vi "Vision Processing.vi"(4 "error in (no error)":errorcluster, 7 "Image Size":T1=enum."320x240") -> ()   [LabVIEW 2016]
doc: "This VI runs in parallel to other tasks. It gets images from the camera, processes them for color or shape and use that information to affect robot behavior."
uses:
  <vilib>/Rock Robotics/WPI/Camera/WPI_CameraImageSize.ctl
  <vilib>/Rock Robotics/WPI/Camera/WPI_CameraWhite Balance Values.ctl
  <vilib>/Rock Robotics/WPI/Camera/WPI_CameraExposure Values.ctl
  <vilib>/Rock Robotics/WPI/Camera/WPI_CameraFrameRate.ctl
  Robot Global Data.vi
panel:
  in  "Image Size 2":T1=enum."320x240"
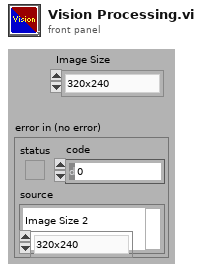
[diagram p1: front panel]
types:
  T1 = typedef "WPI_CameraImageSize.ctl" = enum16{"640x480", "320x240", "160x120", "Custom"}
  T2 = typedef "WPI_CameraFrameRate.ctl" = u32
  T3 = typedef "WPI_CameraExposure Values.ctl" = enum16{"Auto", "Flicker-free 50 Hz", "Flicker-free 60 Hz", "Hold current", "Custom"}
  T4 = typedef "WPI_CameraWhite Balance Values.ctl" = enum16{"Auto", "Fixed indoor", "Fixed outdoor 1", "Fixed outdoor 2", "Fixed fluorescent 1", "Fixed fluorescent 2", "Hold current", "Custom"}
  T5 = typedef "Image Type" = u32
  T6 = typedef "WPI_CameraDevRef.ctl" = cluster{"Camera Address":string, "CameraStatus":errorcluster}
  T7 = typedef "IMAQ Image.ctl" = refnum<image>
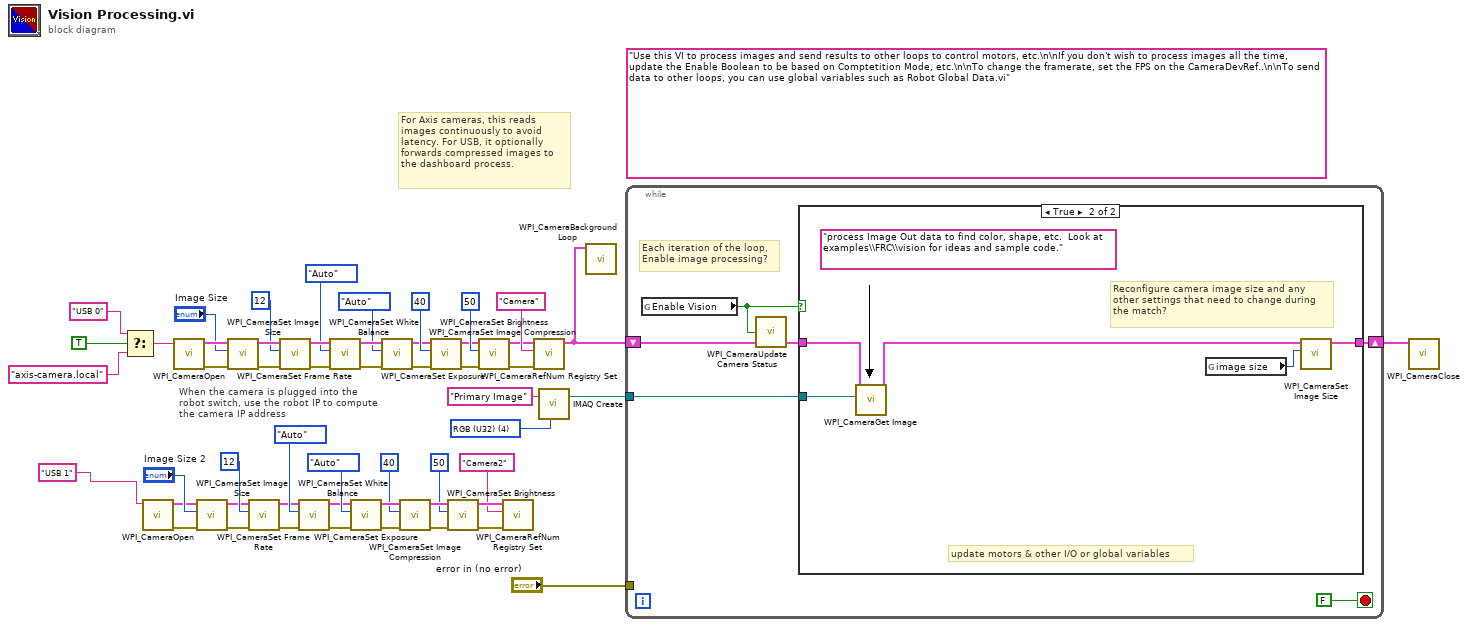
[diagram p0: block diagram]
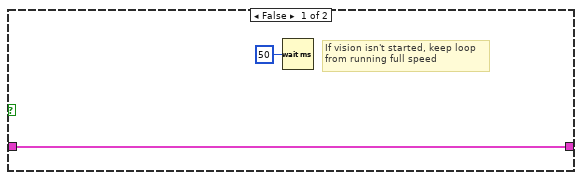
[diagram p2: hidden frame]
diagram:
  (unwired) "Use this VI to process images and send results to other loops to control motors, etc.\n\nIf you don't wish to process images all the time, update the Enable Boolean to be based on Comptetition Mode, etc.\n\nTo change the framerate, set the FPS on the CameraDevRef..\n\nTo send data to other loops, you can use global variables such as Robot Global Data.vi"
  w53 = T5 4 items=["Grayscale (U8)", "Grayscale (I16)", "Grayscale (SGL)", "Complex (CSG)", "RGB (U32)", "HSL (U32)", "RGB (U64)"] ("Image Type")
  # "When the camera is plugged into the\nrobot switch, use the robot IP to compute\nthe camera IP address"
  # "For Axis cameras, this reads\nimages continuously to avoid\nlatency. For USB, it optionally\nforwards compressed images to\nthe dashboard process."
  n1 = Select(t="USB 0" ("format string"), s=TRUE ("dot notation? (F)"), f="axis-camera.local" ("format string")) -> (s? t:f=w24:string)
  n2 = call <vilib>:"WPI_CameraOpen.vi"("Camera Address"="USB 1" ("format string")) -> ("error out"=w11:errorcluster, "CameraDevRef"=w10:T6)  [unwired: 1 in, 8 out]
  n3 = call <vilib>:"WPI_CameraOpen.vi"("Camera Address"=w24) -> ("error out"=w41:errorcluster, "CameraDevRef"=w42:T6)  [unwired: 1 in, 8 out]
  n4 = call <vilib>:"WPI_CameraSet Image Size.vi"("error in (no error)"=w11, "Image Size"="Image Size 2", "CameraDevRef"=w10) -> ("error out"=w12:errorcluster, "CameraDevRef Out"=w9:T6)  [unwired: 1 in, 6 out]
  n5 = call <vilib>:"WPI_CameraSet Image Size.vi"("error in (no error)"=w41, "Image Size"="Image Size", "CameraDevRef"=w42) -> ("error out"=w40:errorcluster, "CameraDevRef Out"=w43:T6)  [unwired: 1 in, 6 out]
  n6 = call <vilib>:"WPI_CameraSet Frame Rate.vi"("error in (no error)"=w12, "Frame Rate (fps)"=T2 12, "CameraDevRef"=w9) -> ("error out"=w13:errorcluster, "CameraDevRef Out"=w7:T6)  [unwired: 7 out]
  n7 = call <vilib>:"WPI_CameraSet Frame Rate.vi"("error in (no error)"=w40, "Frame Rate (fps)"=T2 12, "CameraDevRef"=w43) -> ("error out"=w39:errorcluster, "CameraDevRef Out"=w45:T6)  [unwired: 7 out]
  n8 = call <vilib>:"WPI_CameraSet White Balance.vi"("error in (no error)"=w13, "White Balance"=WPI_CameraWhite_Balance_Values."Auto", "CameraDevRef"=w7) -> ("error out"=w14:errorcluster, "CameraDevRef Out"=w8:T6)  [unwired: 1 in, 6 out]
  n9 = call <vilib>:"WPI_CameraSet White Balance.vi"("error in (no error)"=w39, "White Balance"=WPI_CameraWhite_Balance_Values."Auto", "CameraDevRef"=w45) -> ("error out"=w38:errorcluster, "CameraDevRef Out"=w44:T6)  [unwired: 1 in, 6 out]
  n10 = call <vilib>:"WPI_CameraSet Exposure.vi"("error in (no error)"=w14, "Exposure"=WPI_CameraExposure_Values."Auto", "CameraDevRef"=w8) -> ("error out"=w15:errorcluster, "CameraDevRef Out"=w5:T6)  [unwired: 1 in, 6 out]
  n11 = call <vilib>:"WPI_CameraSet Exposure.vi"("error in (no error)"=w38, "Exposure"=WPI_CameraExposure_Values."Auto", "CameraDevRef"=w44) -> ("error out"=w37:errorcluster, "CameraDevRef Out"=w47:T6)  [unwired: 1 in, 6 out]
  n12 = call <vilib>:"WPI_CameraSet Image Compression.vi"("error in (no error)"=w15, "Compression"=40, "CameraDevRef"=w5) -> ("error out"=w16:errorcluster, "CameraDevRef Out"=w6:T6)  [unwired: 7 out]
  n13 = call <vilib>:"WPI_CameraSet Image Compression.vi"("error in (no error)"=w37, "Compression"=40, "CameraDevRef"=w47) -> ("error out"=w36:errorcluster, "CameraDevRef Out"=w46:T6)  [unwired: 7 out]
  n14 = call <vilib>:"WPI_CameraSet Brightness.vi"("error in (no error)"=w16, "Brightness"=50, "CameraDevRef"=w6) -> ("error out"=w18:errorcluster, "CameraDevRef Out"=w17:T6)  [unwired: 7 out]
  n15 = call <vilib>:"WPI_CameraSet Brightness.vi"("error in (no error)"=w36, "Brightness"=50, "CameraDevRef"=w46) -> ("error out"=w34:errorcluster, "CameraDevRef Out"=w35:T6)  [unwired: 7 out]
  n16 = call <vilib>:"WPI_CameraRefNum Registry Set.vi"("error in (no error)"=w18, "refnum name"="Camera2", "CameraDevRef"=w17) -> ()  [unwired: 1 in, 8 out]
  n17 = call <vilib>:"WPI_CameraRefNum Registry Set.vi"("error in (no error)"=w34, "refnum name"="Camera", "CameraDevRef"=w35) -> ("CameraDevRef"=w30:T6)  [unwired: 1 in, 7 out]
  n18 = call "IMAQ Create"("Image Name"="Primary Image", "Image Type"=w53) -> ("New Image"=w51:T7)  [unwired: 2 in, 2 out]
  n19 = call <vilib>:"WPI_CameraBackground Loop.vi"("CameraDevRef"=w30) -> ()  [unwired: 11 in]
  n20 = while {
    shift-right: [w58] -> w28
    shift-left: w30 -> [w56]
    tunnel: w51 -> [w57]
    tunnel: "error in (no error)" -> [_]
    stop <- FALSE stop-if-true
    # "Each iteration of the loop,\nEnable image processing?"
    n21 = global read "Robot Global Data.vi" "Enable Vision"() -> (w54:bool)
    n22 = call <vilib>:"WPI_CameraUpdate Camera Status.vi"("CameraDevRef In"=w56, "Enable Vision"=w54) -> ("CameraDevRef Out"=w55:T6)  [unwired: 3 in]
    n23 = case shown="True" w54 {
      tunnel: w57 -> [_ w65]
      tunnel: [w61 w66] -> w58
      tunnel: w55 -> [w61 w63]
      frame False {
        # "If vision isn't started, keep loop\nfrom running full speed"
        n24 = Wait (ms)(milliseconds to wait=u32 50) -> ()  [unwired: 1 out]
      }
      frame True {
        (unwired) "process Image Out data to find color, shape, etc.  Look at examples\\FRC\\vision for ideas and sample code."
        # "update motors & other I/O or global variables"
        # "Reconfigure camera image size and any\nother settings that need to change during\nthe match?"
        n25 = call <vilib>:"WPI_CameraGet Image.vi"("Image"=w65, "CameraDevRef"=w63) -> ("CameraDevRef Out"=w62:T6)  [unwired: 1 in, 8 out]
        n26 = global read "Robot Global Data.vi" "image size"() -> (w64:T1)
        n27 = call <vilib>:"WPI_CameraSet Image Size.vi"("Image Size"=w64, "CameraDevRef"=w62) -> ("CameraDevRef Out"=w66:T6)  [unwired: 2 in, 7 out]
      }
    }
  }
  n28 = call <vilib>:"WPI_CameraClose.vi"("CameraDevRef"=w28) -> ()  [unwired: 1 in, 10 out]
